vi "checkQueueFull.vi"(8 "error in (no error)":errorcluster, 10 "queueName":T1(ring), 11 "tcpServerTel in":refnum<class "TcpServerTel.lvclass">) -> (0 "error out":errorcluster, 2 "queueFull":bool, 3 "tcpServerTel out":refnum<class "TcpServerTel.lvclass">)   [LabVIEW 2018, in "TcpServerTel.lvclass"]
doc: "Check if queue is full or not. Use the queueName enum control to select queueTcpClientFromDds or queueTcpClient options."
uses:
  TcpServerTel.lvclass
  home/pcortes/github/ts_labview_tcp_json/src/TcpServerBase/TcpServerBase.lvclass
  TcpServerTel.lvclass/TcpServerTel.ctl
  TcpServerBase/TcpServerBase.lvclass/TcpServerBase.ctl
  TcpServerBase/TcpServerBase.lvclass
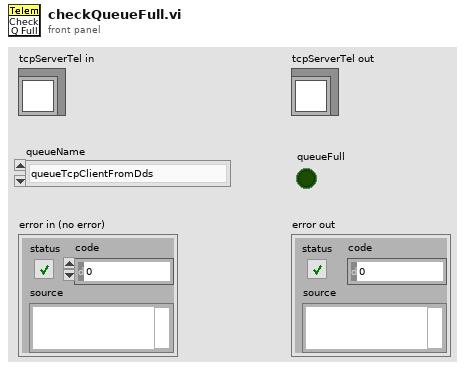
[diagram p1: front panel]
types:
  T1 = enum16{"queueTcpClientFromDds", "queueTcpClient"}
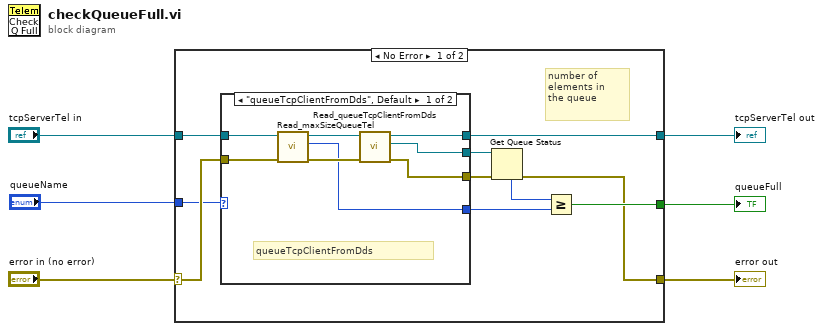
[diagram p0: block diagram]
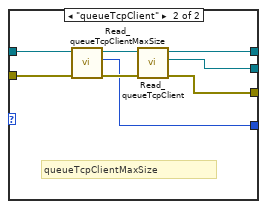
[diagram p2: hidden frame]
diagram:
  n1 = case shown="No Error" "error in (no error)" {
    selector: "error in (no error)" -> [w11 w34]
    tunnel: "tcpServerTel in" -> [w12 w33]
    tunnel: [w10 w33] -> w5
    tunnel: [w8 w34] -> w3
    tunnel: [w9 _] -> w2
    tunnel: "queueName" -> [w7 _]
    frame No Error {
      # "number of\nelements in\nthe queue"
      n2 = case shown="\"queueTcpClientFromDds\", Default" w7 {
        tunnel: [w19 w32] -> w16
        tunnel: [w18 w31] -> w15
        tunnel: [w17 w28] -> w13
        tunnel: w12 -> [w24 w27]
        tunnel: w11 -> [w21 w26]
        tunnel: [w22 w25] -> w10
        frame "queueTcpClientFromDds", Default {
          # "queueTcpClientFromDds"
          n3 = call "Read_maxSizeQueueTel.vi"("error in (no error)"=w21, "TcpServerTel in"=w24) -> ("error out"=w20:errorcluster, "maxSizeQueueTel"=w17:i32, "TcpServerTel out"=w23:refnum<class "TcpServerTel.lvclass">)  [unwired: 7 in]
          n4 = call "Read_queueTcpClientFromDds.vi"("error in (no error)"=w20, "TcpServerTel in"=w23) -> ("error out"=w19:errorcluster, "queueTcpClientFromDds"=w18:refnum<queue>, "TcpServerTel out"=w22:refnum<class "TcpServerTel.lvclass">)  [unwired: 7 in]
        }
        frame "queueTcpClient" {
          # "queueTcpClientMaxSize"
          n5 = call "Read_queueTcpClientMaxSize.vi"("error in (no error)"=w26, "TcpServerBase in"=w27) -> ("error out"=w30:errorcluster, "queueTcpClientMaxSize"=w28:i32, "TcpServerBase out"=w29:refnum<class "TcpServerTel.lvclass">)  [unwired: 7 in]
          n6 = call "Read_queueTcpClient.vi"("error in (no error)"=w30, "TcpServerBase in"=w29) -> ("error out"=w32:errorcluster, "queueTcpClient"=w31:refnum<queue>, "TcpServerBase out"=w25:refnum<class "TcpServerTel.lvclass">)  [unwired: 7 in]
        }
      }
      n7 = Get Queue Status(queue=w15, error in (no error)=w16) -> (error out=w8:errorcluster, # elements in queue=w14:i32)  [unwired: 1 in, 6 out]
      n8 = Greater Or Equal?(x=w14, y=w13) -> (x >= y?=w9:bool)
    }
    frame Error {
    }
  }
  "error out" <- w3
  "tcpServerTel out" <- w5
  "queueFull" <- w2
